vi "robotOrientatedToBall.vi"(8 "error in (no error)":errorcluster, 9 "Robot":refnum<class "Robot.lvclass">, 10 "BallRef":refnum<class "Ball.lvclass">, 11 "Utilities in":refnum<class "Utilities.lvclass">) -> (0 "error out":errorcluster, 2 "Orientation":dbl, 3 "Utilities out":refnum<class "Utilities.lvclass">)   [LabVIEW 2023, in "Utilities.lvclass"]
uses:
  Utilities.lvclass
  Robot_class/Robot.lvclass
  Ball_class/Ball.lvclass
  Object_class/Object.lvclass/Object.ctl
  Object_class/Read x.vi
  Object_class/Read y.vi
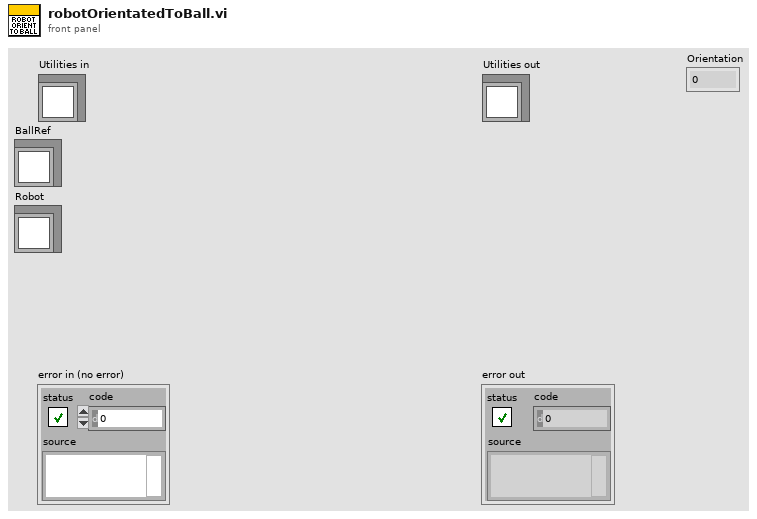
[diagram p1: front panel]
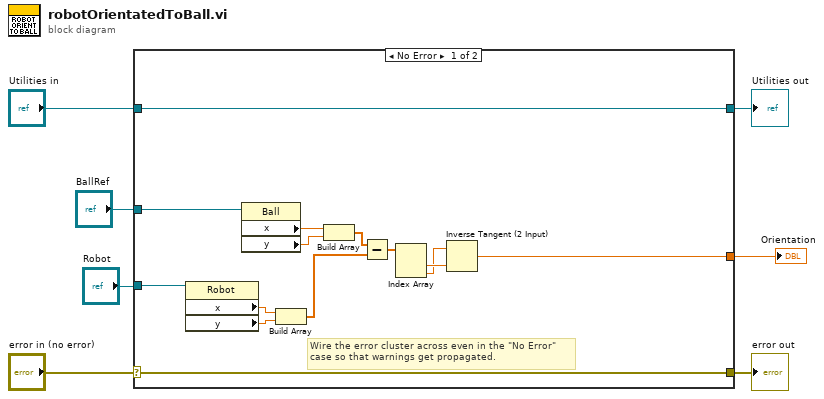
[diagram p0: block diagram]
diagram:
  n1 = case shown="No Error" "error in (no error)" {
    selector: "error in (no error)" -> [w20 w23]
    tunnel: [w20 w23] -> w6
    tunnel: [w21 w22] -> w4
    tunnel: "Utilities in" -> [w21 w22]
    tunnel: "Robot" -> [w16 _]
    tunnel: [w9 _] -> w2
    tunnel: "BallRef" -> [w8 _]
    frame No Error {
      # "Wire the error cluster across even in the \"No Error\"\ncase so that warnings get propagated."
      n2 = property class="Robot"(reference=w16) -> ("x"=w15:dbl, "y"=w14:dbl)  [unwired: 1 in, 2 out]
      n3 = property class="Ball"(reference=w8) -> ("x"=w19:dbl, "y"=w18:dbl)  [unwired: 1 in, 2 out]
      n4 = Build Array(w15, w14) -> (w13:dbl[])
      n5 = Build Array(w19, w18) -> (w17:dbl[])
      n6 = Subtract(x=w17, y=w13) -> (x-y=w12:dbl[])
      n7 = Index Array(array=w12) -> (element #1=w11:dbl, element #2=w10:dbl)  [unwired: 2 in]
      n8 = Inverse Tangent (2 Input)(1:w11, 2:w10) -> (0:w9:dbl)
    }
    frame Error {
    }
  }
  "error out" <- w6
  "Utilities out" <- w4
  "Orientation" <- w2
